vi "LessThanBasicExample.vi"() -> ()   [LabVIEW 2013]
panel:
  out "Device Status":i32 format="%x"
  in  "stop":bool
  out "DeviceInfo":T1
  in  "resource name":refnum<visa-resource-name>
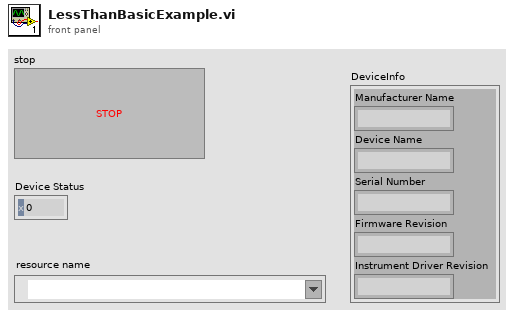
[diagram p1: front panel]
types:
  T1 = cluster{"Manufacturer Name":string, "Device Name":string, "Serial Number":string, "Firmware Revision":string, "Instrument Driver Revision":string}
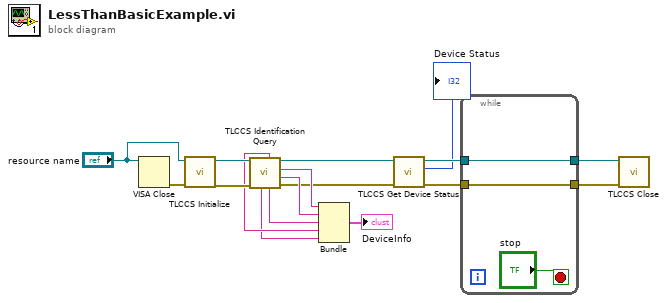
[diagram p0: block diagram]
diagram:
  n1 = VISA Close(VISA resource name="resource name") -> (error out=w17:errorcluster)  [unwired: 1 in]
  n2 = call <instrlib>:"TLCCS Initialize.vi"("error in (no error)"=w17, "resource name"="resource name") -> ("error out"=w15:errorcluster, "instrument handle out"=w14:refnum<visa-resource-name>)  [unwired: 8 in]
  n3 = call <instrlib>:"TLCCS Identification Query.vi"("error in (no error)"=w15, "instrument handle"=w14) -> ("error out"=w7:errorcluster, "Device Name"=w12:string, "Manufacturer Name"=w13:string, "instrument handle out"=w6:refnum<visa-resource-name>, "Serial Number"=w11:string, "Firmware Revision"=w10:string, "Instrument Driver Revision"=w9:string)  [unwired: 3 in]
  n4 = Bundle("Manufacturer Name"=w13, "Device Name"=w12, "Serial Number"=w11, "Firmware Revision"=w10, "Instrument Driver Revision"=w9) -> (→"DeviceInfo":T1)  [unwired: 1 in]
  n5 = call <instrlib>:"TLCCS Get Device Status.vi"("error in (no error)"=w7, "instrument handle"=w6) -> ("error out"=w4:errorcluster, "Device Status"=→"Device Status":i32, "instrument handle out"=w3:refnum<visa-resource-name>)  [unwired: 7 in]
  n6 = while {
    tunnel: [w20] -> w5
    tunnel: w4 -> [w20]
    tunnel: [w19] -> w2
    tunnel: w3 -> [w19]
    stop <- "stop" stop-if-true
  }
  n7 = call <instrlib>:"TLCCS Close.vi"("error in (no error)"=w5, "instrument handle"=w2) -> ()  [unwired: 9 in, 1 out]
